vi "Verificar Credito.vi"(7 "STOP":bool=TRUE, 8 "error in (no error)":errorcluster, 9 "Credito":i32, 10 "Servicio":string, 11 "UI in":refnum<class "UI.lvclass">) -> (0 "error out":errorcluster, 3 "UI out":refnum<class "UI.lvclass">)   [LabVIEW 2020, in "UI.lvlib" / "UI.lvclass"]
uses:
  UI.lvclass
  UI.lvclass/UI.ctl
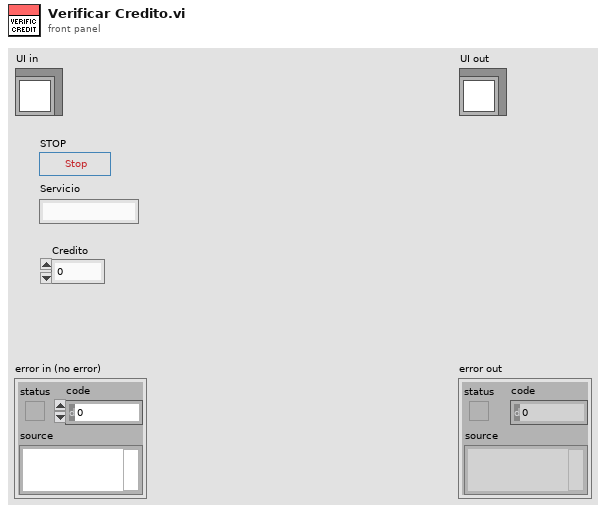
[diagram p1: front panel]
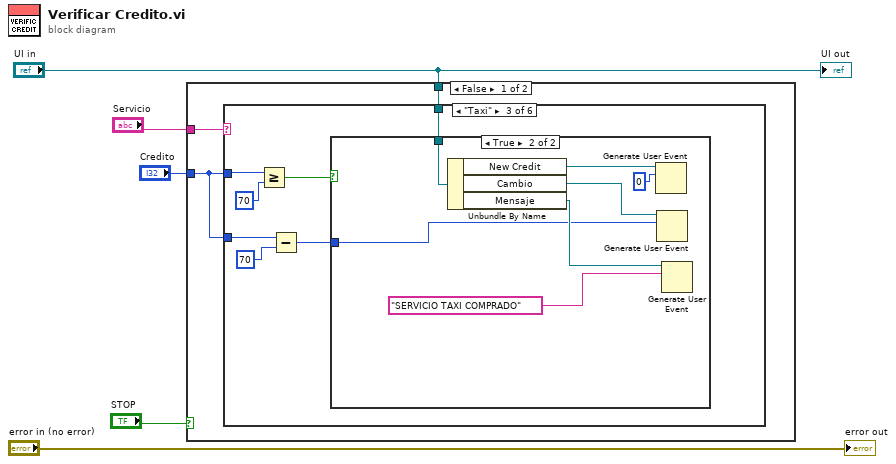
[diagram p0: block diagram]
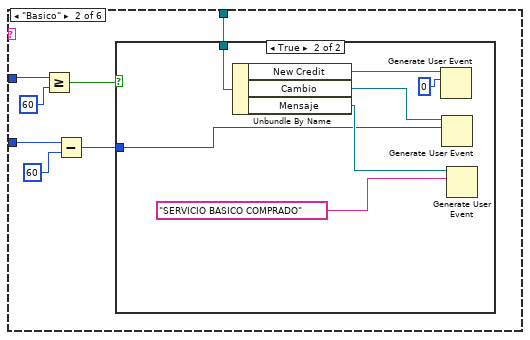
[diagram p3: hidden frame]
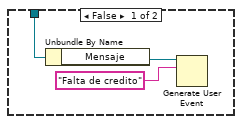
[diagram p4: hidden frame]
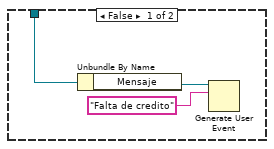
[diagram p5: hidden frame]
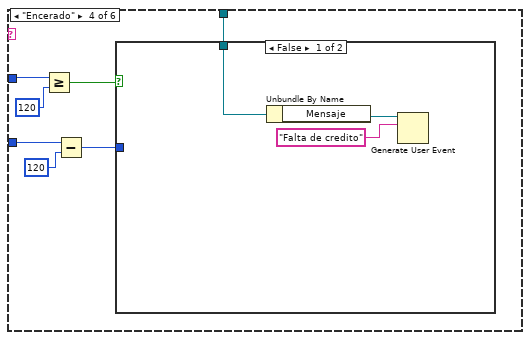
[diagram p6: hidden frame]
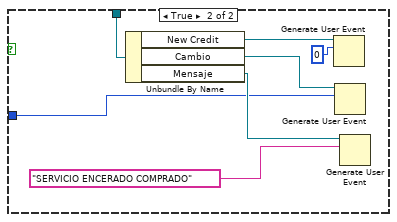
[diagram p7: hidden frame]
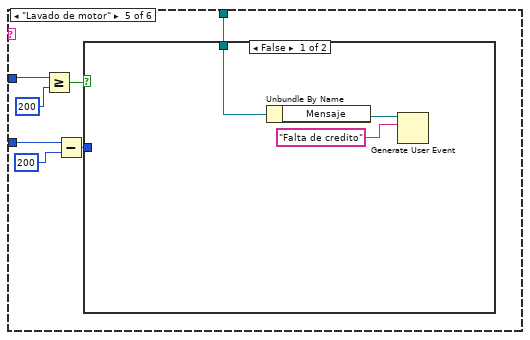
[diagram p8: hidden frame]
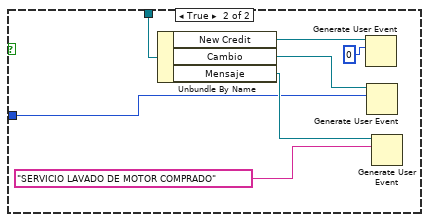
[diagram p9: hidden frame]
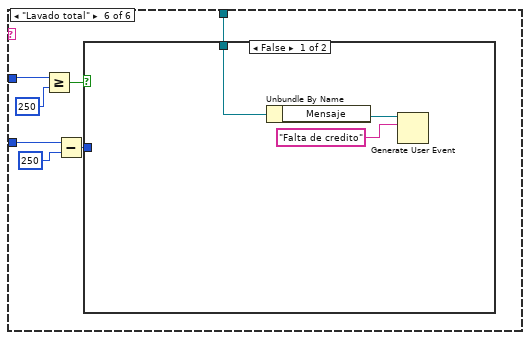
[diagram p10: hidden frame]
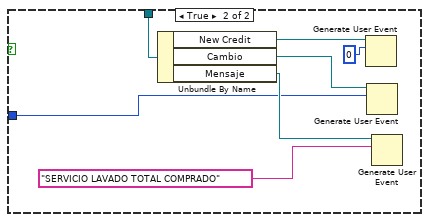
[diagram p11: hidden frame]
diagram:
  n1 = case shown="False" "STOP" {
    tunnel: "Servicio" -> [w6 _]
    tunnel: "Credito" -> [w8 _]
    tunnel: "UI in" -> [w7 _]
    frame False {
      n2 = case shown="\"Taxi\"" w6 {
        tunnel: w8 -> [_ w15 w32 w49 w66 w83]
        tunnel: w8 -> [_ w10 w27 w43 w61 w78]
        tunnel: w7 -> [_ w11 w28 w45 w62 w79]
        frame Default {
        }
        frame "Basico" {
          n3 = Greater Or Equal?(x=w15, y=60) -> (x >= y?=w14:bool)
          n4 = Subtract(x=w10, y=60 ("x")) -> (x-y=w12:i32)
          n5 = case shown="True" w14 {
            tunnel: w12 -> [_ w20]
            tunnel: w11 -> [w18 w25]
            frame False {
              n6 = Unbundle By Name(w18) -> ("Mensaje"=w17:refnum<user-event>)
              n7 = Generate User Event(user event=w17, event data cluster="Falta de credito" ("event data")) -> ()  [unwired: 2 in, 2 out]
            }
            frame True {
              n8 = Unbundle By Name(w25) -> ("New Credit"=w24:refnum<user-event>, "Cambio"=w23:refnum<user-event>, "Mensaje"=w22:refnum<user-event>)
              n9 = Generate User Event(user event=w24, event data cluster=0 ("event data")) -> ()  [unwired: 2 in, 2 out]
              n10 = Generate User Event(user event=w23, event data cluster=w20) -> ()  [unwired: 2 in, 2 out]
              n11 = Generate User Event(user event=w22, event data cluster="SERVICIO BASICO COMPRADO" ("event data")) -> ()  [unwired: 2 in, 2 out]
            }
          }
        }
        frame "Taxi" {
          n12 = Greater Or Equal?(x=w32, y=70) -> (x >= y?=w31:bool)
          n13 = Subtract(x=w27, y=70 ("x")) -> (x-y=w29:i32)
          n14 = case shown="True" w31 {
            tunnel: w29 -> [_ w37]
            tunnel: w28 -> [w33 w42]
            frame False {
              n15 = Unbundle By Name(w33) -> ("Mensaje"=w35:refnum<user-event>)
              n16 = Generate User Event(user event=w35, event data cluster="Falta de credito" ("event data")) -> ()  [unwired: 2 in, 2 out]
            }
            frame True {
              n17 = Unbundle By Name(w42) -> ("New Credit"=w41:refnum<user-event>, "Cambio"=w40:refnum<user-event>, "Mensaje"=w39:refnum<user-event>)
              n18 = Generate User Event(user event=w41, event data cluster=0 ("event data")) -> ()  [unwired: 2 in, 2 out]
              n19 = Generate User Event(user event=w40, event data cluster=w37) -> ()  [unwired: 2 in, 2 out]
              n20 = Generate User Event(user event=w39, event data cluster="SERVICIO TAXI COMPRADO" ("event data")) -> ()  [unwired: 2 in, 2 out]
            }
          }
        }
        frame "Encerado" {
          n21 = Greater Or Equal?(x=w49, y=120) -> (x >= y?=w48:bool)
          n22 = Subtract(x=w43, y=120 ("x")) -> (x-y=w46:i32)
          n23 = case shown="False" w48 {
            tunnel: w46 -> [_ w54]
            tunnel: w45 -> [w50 w59]
            frame False {
              n24 = Unbundle By Name(w50) -> ("Mensaje"=w52:refnum<user-event>)
              n25 = Generate User Event(user event=w52, event data cluster="Falta de credito" ("event data")) -> ()  [unwired: 2 in, 2 out]
            }
            frame True {
              n26 = Unbundle By Name(w59) -> ("New Credit"=w58:refnum<user-event>, "Cambio"=w57:refnum<user-event>, "Mensaje"=w56:refnum<user-event>)
              n27 = Generate User Event(user event=w58, event data cluster=0 ("event data")) -> ()  [unwired: 2 in, 2 out]
              n28 = Generate User Event(user event=w57, event data cluster=w54) -> ()  [unwired: 2 in, 2 out]
              n29 = Generate User Event(user event=w56, event data cluster="SERVICIO ENCERADO COMPRADO" ("event data")) -> ()  [unwired: 2 in, 2 out]
            }
          }
        }
        frame "Lavado de motor" {
          n30 = Greater Or Equal?(x=w66, y=200) -> (x >= y?=w65:bool)
          n31 = Subtract(x=w61, y=200 ("x")) -> (x-y=w63:i32)
          n32 = case shown="False" w65 {
            tunnel: w63 -> [_ w71]
            tunnel: w62 -> [w67 w76]
            frame False {
              n33 = Unbundle By Name(w67) -> ("Mensaje"=w69:refnum<user-event>)
              n34 = Generate User Event(user event=w69, event data cluster="Falta de credito" ("event data")) -> ()  [unwired: 2 in, 2 out]
            }
            frame True {
              n35 = Unbundle By Name(w76) -> ("New Credit"=w75:refnum<user-event>, "Cambio"=w74:refnum<user-event>, "Mensaje"=w73:refnum<user-event>)
              n36 = Generate User Event(user event=w75, event data cluster=0 ("event data")) -> ()  [unwired: 2 in, 2 out]
              n37 = Generate User Event(user event=w74, event data cluster=w71) -> ()  [unwired: 2 in, 2 out]
              n38 = Generate User Event(user event=w73, event data cluster="SERVICIO LAVADO DE MOTOR COMPRADO" ("event data")) -> ()  [unwired: 2 in, 2 out]
            }
          }
        }
        frame "Lavado total" {
          n39 = Greater Or Equal?(x=w83, y=250) -> (x >= y?=w82:bool)
          n40 = Subtract(x=w78, y=250 ("x")) -> (x-y=w80:i32)
          n41 = case shown="False" w82 {
            tunnel: w80 -> [_ w88]
            tunnel: w79 -> [w84 w93]
            frame False {
              n42 = Unbundle By Name(w84) -> ("Mensaje"=w86:refnum<user-event>)
              n43 = Generate User Event(user event=w86, event data cluster="Falta de credito" ("event data")) -> ()  [unwired: 2 in, 2 out]
            }
            frame True {
              n44 = Unbundle By Name(w93) -> ("New Credit"=w92:refnum<user-event>, "Cambio"=w91:refnum<user-event>, "Mensaje"=w90:refnum<user-event>)
              n45 = Generate User Event(user event=w92, event data cluster=0 ("event data")) -> ()  [unwired: 2 in, 2 out]
              n46 = Generate User Event(user event=w91, event data cluster=w88) -> ()  [unwired: 2 in, 2 out]
              n47 = Generate User Event(user event=w90, event data cluster="SERVICIO LAVADO TOTAL COMPRADO" ("event data")) -> ()  [unwired: 2 in, 2 out]
            }
          }
        }
      }
    }
    frame True {
    }
  }
  "error out" <- "error in (no error)"
  "UI out" <- "UI in"
